vi "LCR.vi"(8 "Error In":errorcluster, 10 "Function":T1=16 items=["Cs-Q", "Cs-D", "Cs-R", "Cp-Q", "Cp-D", "Cp-R", "Cp-G", "Ls-Q", "Ls-D", "Ls-R", "Lp-Q", "Lp-D", "Lp-R", "Lp-G", "Z-th", "Y-th", "R-X", "G-B", "DCR"], 11 "LCR":T2) -> (0 "Error Out":errorcluster, 1 "Measured Secondary Reading":dbl, 2 "Measured Primary Reading":dbl)   [LabVIEW 2018]
uses:
  controls/LCR.ctl
  controls/LCR function.ctl
  <instrlib>/BK Precision 891/BK Precision 891.lvlib
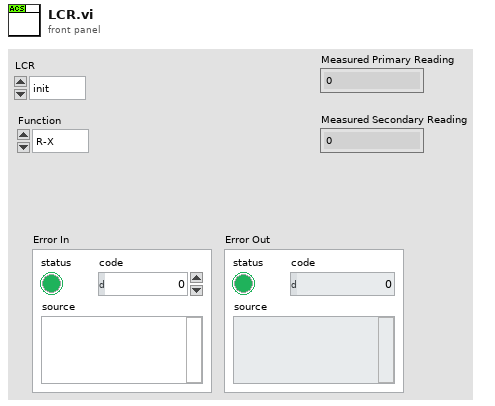
[diagram p1: front panel]
types:
  T1 = typedef "LCR function.ctl" = u16
  T2 = typedef "LCR.ctl" = enum16{"init", "config measurement", "config measurement signal", "read measurement", "close"}
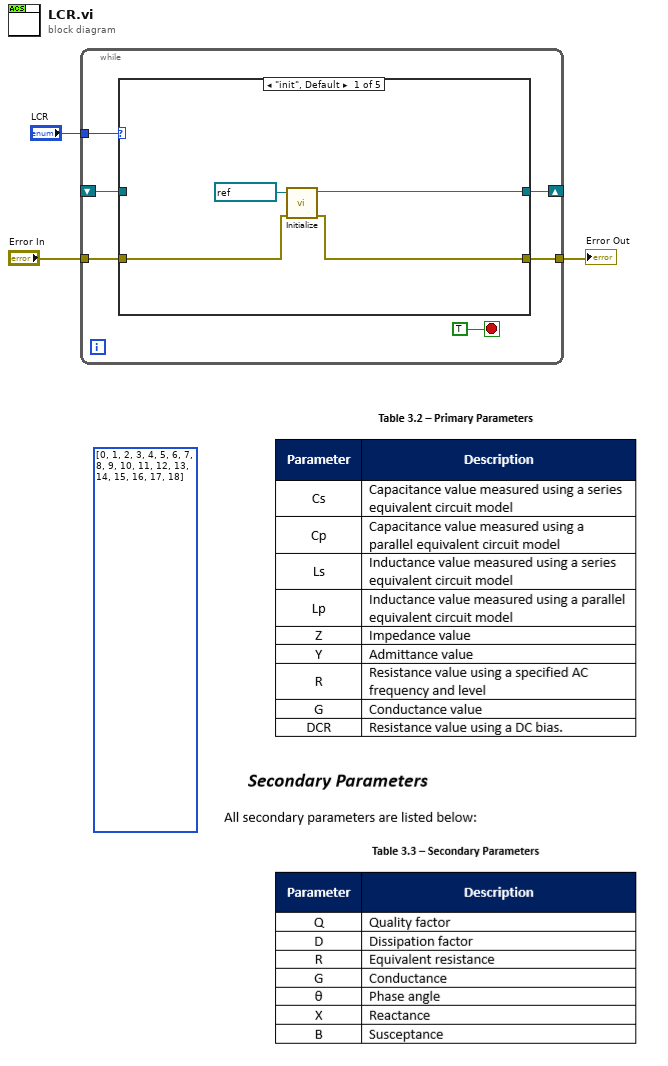
[diagram p0: block diagram]
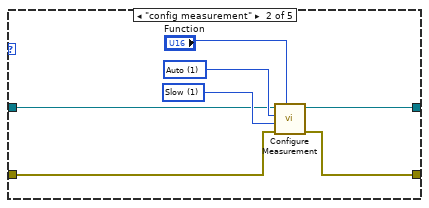
[diagram p2: hidden frame]
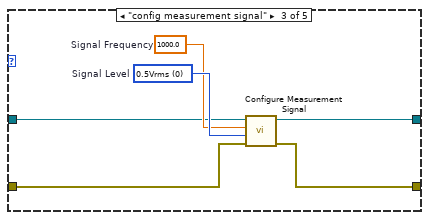
[diagram p3: hidden frame]
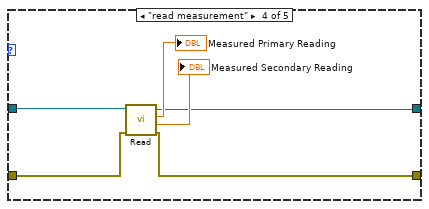
[diagram p4: hidden frame]
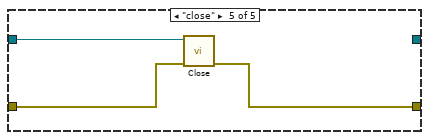
[diagram p5: hidden frame]
diagram:
  (unwired) T1[] [0, 1, 2, 3, 4, 5, 6, 7, 8, 9, 10, 11, 12, 13, 14, 15, 16, 17, 18] items=["Cs-Q", "Cs-D", "Cs-R", "Cp-Q", "Cp-D", "Cp-R", "Cp-G", "Ls-Q", "Ls-D", "Ls-R", "Lp-Q", "Lp-D", "Lp-R", "Lp-G", "Z-th", "Y-th", "R-X", "G-B", "DCR"]
  n1 = while {
    tunnel: "LCR" -> [w9]
    shift-right: [w7] -> _
    shift-left: _ -> [w6]
    tunnel: "Error In" -> [w5]
    tunnel: [w4] -> w1
    stop <- TRUE stop-if-true
    n2 = case shown="\"init\", Default" w9 {
      tunnel: [w12 w16 w23 w28 _] -> w7
      tunnel: w6 -> [_ w17 w24 w30 w35]
      tunnel: w5 -> [w11 w15 w22 w29 w34]
      tunnel: [w10 w14 w21 w27 w33] -> w4
      frame "init", Default {
        n3 = call <instrlib>:"Initialize.vi"("error in (no error)"=w11, "VISA resource name"=refnum<visa-resource-name> "COM3") -> ("error out"=w10:errorcluster, "VISA resource name out"=w12:refnum<visa-resource-name>)  [unwired: 8 in]
      }
      frame "config measurement" {
        w19 = u16 1 items=["Slow"=1, "Fast"=2] ("Measurement Speed")
        w20 = u16 1 items=["Hold", "Auto"] ("Range")
        n4 = call <instrlib>:"Configure Measurement.vi"("Function (4: Cp-D)"="Function", "error in (no error)"=w15, "Measurement Speed (2:Fast)"=w19, "Range (1:Auto)"=w20, "VISA resource name"=w17) -> ("error out"=w14:errorcluster, "VISA resource name out"=w16:refnum<visa-resource-name>)  [unwired: 5 in]
      }
      frame "config measurement signal" {
        w26 = u8 0 items=["0.5Vrms", "1Vrms"]  # Signal Level
        w25 = 1000.0  # Signal Frequency
        n5 = call <instrlib>:"Configure Measurement Signal.vi"("error in (no error)"=w22, "Signal Level (0:0.5 Vrms)"=w26, "Signal Frequency (1000 Hz)"=w25, "VISA resource name"=w24) -> ("error out"=w21:errorcluster, "VISA resource name out"=w23:refnum<visa-resource-name>)  [unwired: 6 in]
      }
      frame "read measurement" {
        n6 = call <instrlib>:"Read.vi"("error in (no error)"=w29, "VISA resource name"=w30) -> ("error out"=w27:errorcluster, "Measured Secondary Reading"=→"Measured Secondary Reading":dbl, "Measured Primary Reading"=→"Measured Primary Reading":dbl, "VISA resource name out"=w28:refnum<visa-resource-name>)  [unwired: 6 in]
      }
      frame "close" {
        n7 = call <instrlib>:"Close.vi"("error in (no error)"=w34, "VISA resource name"=w35) -> ("error out"=w33:errorcluster)  [unwired: 9 in]
      }
    }
  }
  "Error Out" <- w1
